vi "GetFlowRate.vi"(8 "Error In":errorcluster, 11 "Sierra M100 In":refnum<visa-resource-name>) -> (0 "Error Out":errorcluster, 1 "Flow Rate Found?":bool, 2 "Flow Rate":dbl format="%.1f", 3 "Sierra M100 Out":refnum<visa-resource-name>)   [LabVIEW 2012, in "Sierra-M100.lvlib"]
doc: "This VI gets the flow rate from the mass flow controller (MFC). Use the \"Get Units\" VI to determine the units of the return value."
uses:
  Sierra-M100.lvlib
  <vilib>/regexp/Match Regular Expression.xnode
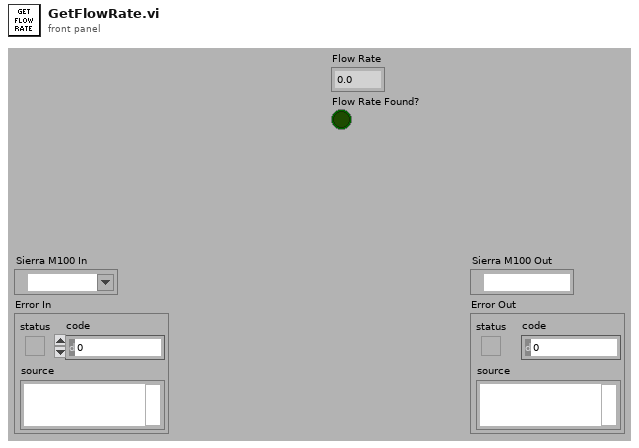
[diagram p1: front panel]
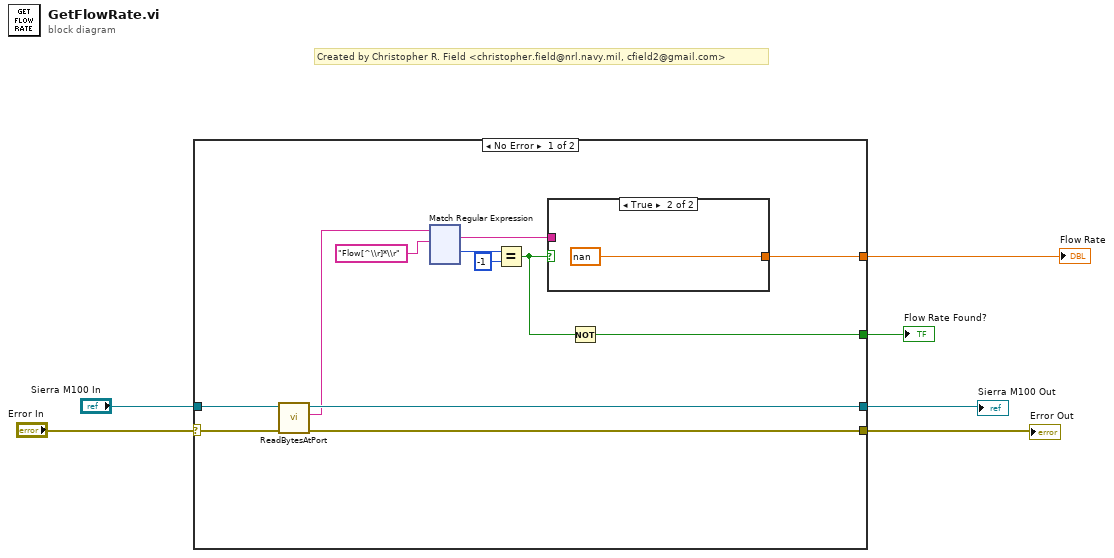
[diagram p0: block diagram]
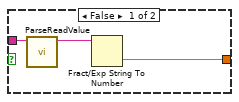
[diagram p2: hidden frame]
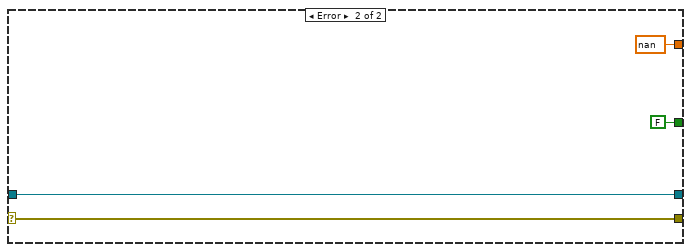
[diagram p3: hidden frame]
diagram:
  # "Created by Christopher R. Field <christopher.field@nrl.navy.mil, cfield2@gmail.com>"
  n1 = case shown="No Error" "Error In" {
    selector: "Error In" -> [w7 w137]
    tunnel: [w18 w136] -> w6
    tunnel: [w17 w137] -> w5
    tunnel: "Sierra M100 In" -> [w16 w136]
    tunnel: [w10 nan] -> w3
    tunnel: [w8 FALSE] -> w2
    frame No Error {
      n2 = call "ReadBytesAtPort.vi"("Error In"=w7, "Smart Trak 2 In"=w16) -> ("Error Out"=w17:errorcluster, "Read Buffer"=w14:string, "Smart Trak 2 Out"=w18:refnum<visa-resource-name>)  [unwired: 7 in]
      n3 = xnode "Match Regular Expression"("input string"=w14, "regular expression"="Flow[^\\r]*\\r" ("string")) -> ("whole match"=w13:string, "offset past match"=w12:i32)  [unwired: 4 in, 3 out]
      n4 = Equal?(x=w12, y=-1) -> (x = y?=w9:bool)
      n5 = case shown="True" w9 {
        tunnel: w13 -> [w21 _]
        tunnel: [w19 nan] -> w10
        frame False {
          n6 = call "ParseReadValue.vi"("Read Buffer"=w21) -> ("Value"=w20:string)  [unwired: 10 in]
          n7 = Fract/Exp String To Number(string=w20) -> (number=w19:dbl)  [unwired: 3 in, 1 out]
        }
        frame True {
        }
      }
      n8 = Not(x=w9) -> (.not. x?=w8:bool)
    }
    frame Error {
    }
  }
  "Sierra M100 Out" <- w6
  "Error Out" <- w5
  "Flow Rate" <- w3
  "Flow Rate Found?" <- w2
